vi "setBit.vi"(10 "n":i32=-1, 11 "input":u8 format="%08b") -> (3 "output":u8 format="%08b")   [LabVIEW 2013, in "bitwiseOps.lvlib"]
uses:
  bitwiseOps.lvlib
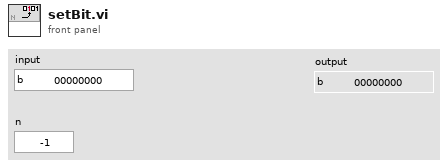
[diagram p1: front panel]
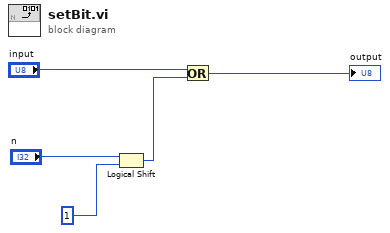
[diagram p0: block diagram]
diagram:
  n1 = Logical Shift(y="n", x=u8 1) -> (x << y=w4:u8)
  n2 = Or(x="input", y=w4) -> (x .or. y?=→"output":u8)
